vi "DecodeRS232 Message.vi"() -> ()   [LabVIEW 2014]
panel:
  in  "8 bit CRC Checksum?":bool
  in  "RS232 Sentence Input":string
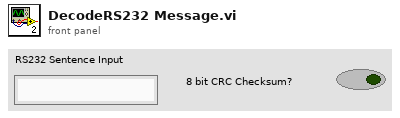
[diagram p1: front panel]
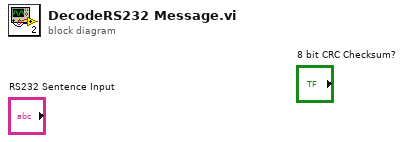
[diagram p0: block diagram]
diagram:
